vi "ImageRecon-Mov cor.vi"(7 "Logging queue element in":T1={"Imaging Protocol"=enum."Live Imaging", "Number of Trials"=0, "Frame Size"=512, "# Averaged frames"=0, "Dwell time (us)"=0.0, "Index of Z-plane"=0, "Timelapse?"=FALSE, "Logging process is active"=FALSE, "Speed logging enabled"=FALSE, "tdms file ref"=refnum, "path"=path "", "Trial Number"=0, "Expected # points acquired"=FALSE, "Manually stopped"=FALSE, "Ch0 data"=[], "Ch1 data"=[], "Ref Data"=[], "Last trial"=FALSE, "Ref Dwell time (us)"=0.0, "# Ref Averaged frames"=0, "Ref X Length"=0, "Ref Y Length"=0, "Points acquired"={"Ch0 last trial"=0, "Ch1 last trial"=0, "All trials"=0}} {"Ref Dwell time (us)" format="%#.6g"; "Frame Size" items=["100X100"=100, "128X128"=128, "200X200"=200, "256X256"=256, "512X512"=512, "1024x1024"=1024, "2048x2048"=2048]; "Dwell time (us)" format="%#.6g"}, 8 "Error In":errorcluster, 9 "Data":T5, 11 "Image Array (in)":T6) -> (0 "Error Out":errorcluster, 1 "Ch1-Green-REF":i16[][](graph), 2 "Ch0-Red-REF":i16[][](graph), 3 "Image Array(out)":T6)   [LabVIEW 2017]
uses:
  Queue/Live graphs queue/Typedefs/Live imaging queue element.ctl
  <vilib>/vision/Image Controls.llb/IMAQ Image.ctl
  Typedefs/Frame data dual cluster.ctl
  Typedefs/Logging queue element.ctl
  Typedefs/Imaging Protocols enum.ctl
  Typedefs/Frame Size.ctl
  Typedefs/Acquired points count.ctl
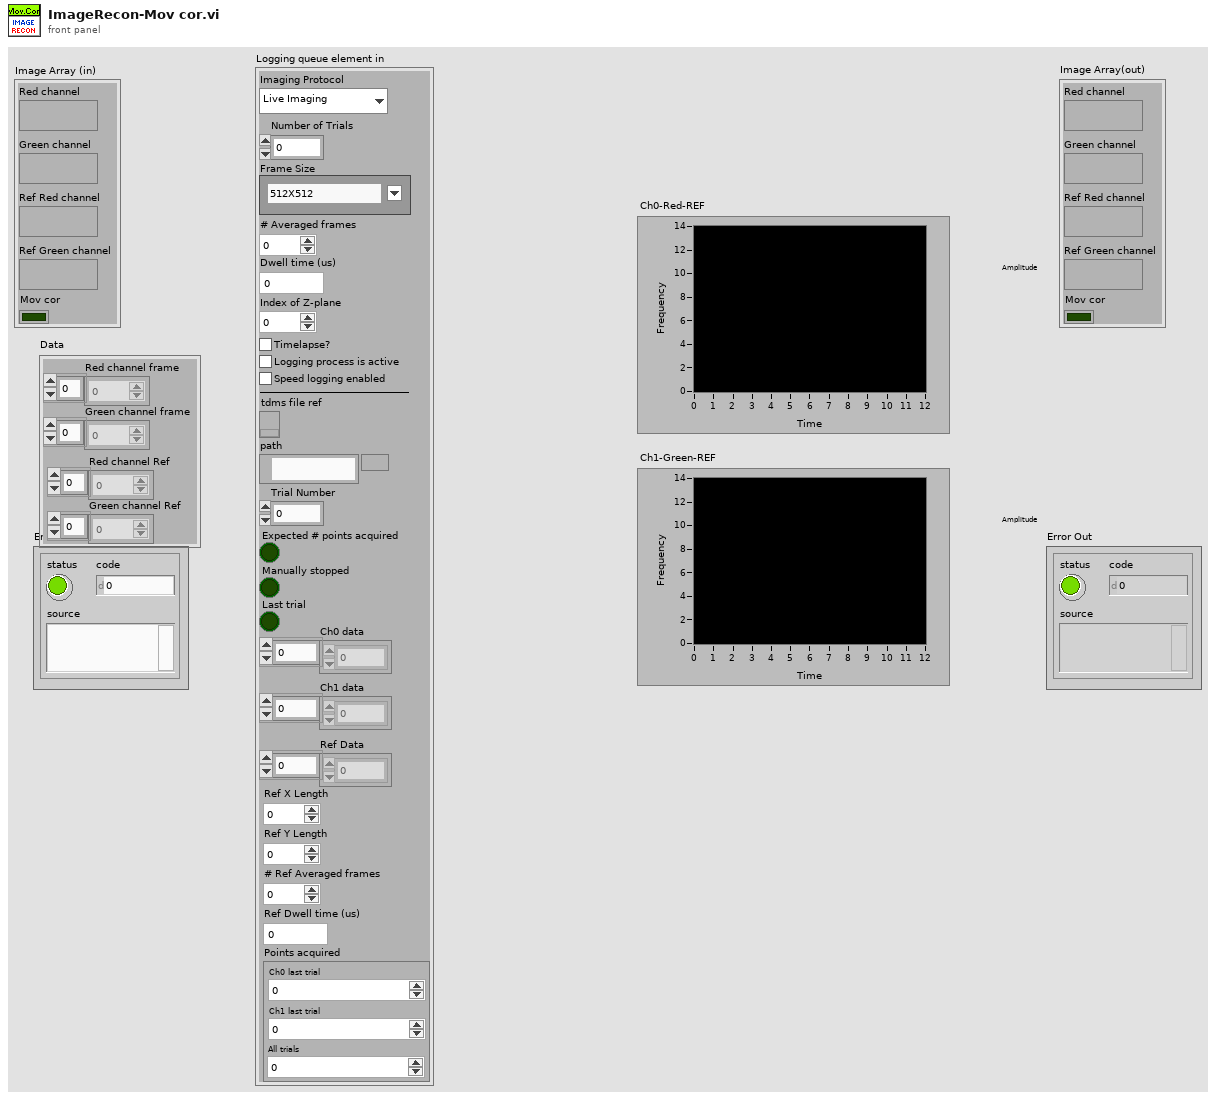
[diagram p1: front panel]
types:
  T1 = typedef "Logging queue element.ctl" = cluster{"Imaging Protocol":T2, "Number of Trials":u16, "Frame Size":T3, "# Averaged frames":u16, "Dwell time (us)":dbl, "Index of Z-plane":i32, "Timelapse?":bool, "Logging process is active":bool, "Speed logging enabled":bool, "tdms file ref":refnum<k34>, "path":path, "Trial Number":i32, "Expected # points acquired":bool, "Manually stopped":bool, "Ch0 data":u32[], "Ch1 data":u32[], "Ref Data":u32[], "Last trial":bool, "Ref Dwell time (us)":dbl, "# Ref Averaged frames":u16, "Ref X Length":u16, "Ref Y Length":u16, "Points acquired":T4}
  T2 = typedef "Imaging Protocols enum.ctl" = enum16{"AOL Z-Stack", "Motor Z Stack", "Functional Acquisition", "Single Plane Acquisition", "Volume Acquisition", "Live Imaging", "Live Plane Imaging", "Live Volume Imaging"}
  T3 = typedef "Frame Size.ctl" = u16
  T4 = typedef "Acquired points count.ctl" = cluster{"Ch0 last trial":u64, "Ch1 last trial":u64, "All trials":u64}
  T5 = typedef "Frame data dual cluster.ctl" = cluster{"Red channel frame":dbl[], "Green channel frame":dbl[], "Red channel Ref":dbl[], "Green channel Ref":dbl[]}
  T6 = typedef "Live imaging queue element.ctl" = cluster{"Red channel":T7, "Green channel":T7, "Ref Red channel":T7, "Ref Green channel":T7, "Mov cor":bool}
  T7 = typedef "IMAQ Image.ctl" = refnum<image>
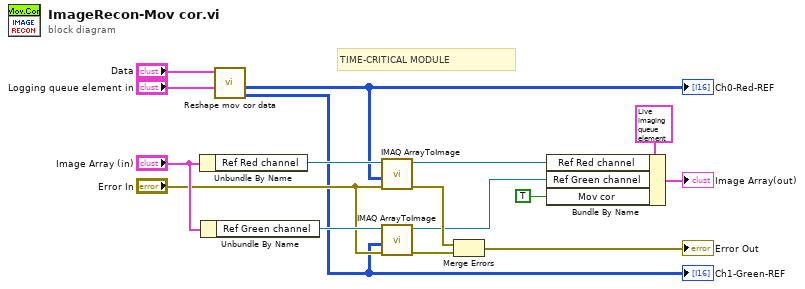
[diagram p0: block diagram]
diagram:
  # "TIME-CRITICAL MODULE"
  n1 = Unbundle By Name("Image Array (in)") -> ("Ref Red channel"=w13:T7)
  n2 = Unbundle By Name("Image Array (in)") -> ("Ref Green channel"=w10:T7)
  n3 = call "Reshape mov cor data.vi"("Logging queue element in"="Logging queue element in", "Data"="Data") -> ("Ch1- Green Ref"=w5:i16[][], "Ch0-Red Ref"=w1:i16[][])  [unwired: 8 in]
  "Ch0-Red-REF" <- w1
  "Ch1-Green-REF" <- w5
  n4 = call "IMAQ ArrayToImage"("error in (no error)"="Error In", "Image Pixels (I16)"=w1, "Image"=w13) -> ("error out"=w15:errorcluster, "Image Out"=w3:T7)  [unwired: 7 in]
  n5 = call "IMAQ ArrayToImage"("error in (no error)"="Error In", "Image Pixels (I16)"=w5, "Image"=w10) -> ("error out"=w14:errorcluster, "Image Out"=w2:T7)  [unwired: 7 in]
  n6 = Merge Errors(w15, w14) -> (→"Error Out":errorcluster)
  n7 = Bundle By Name(cluster=T6 {"Red channel"=refnum, "Green channel"=refnum, "Ref Red channel"=refnum, "Ref Green channel"=refnum, "Mov cor"=FALSE} ("Image Array(out)"), "Ref Red channel"=w3, "Ref Green channel"=w2, "Mov cor"=TRUE) -> (→"Image Array(out)":T6)
